vi "TempStringFormatter.vi"(11 "Parsed List":string[](array[string])) -> (3 "string to write":string)   [LabVIEW 2012]
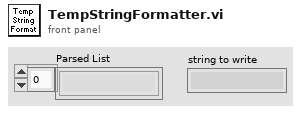
[diagram p1: front panel]
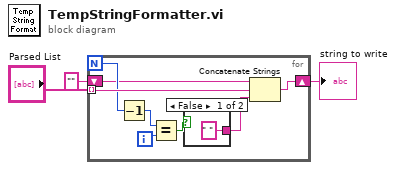
[diagram p0: block diagram]
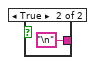
[diagram p2: hidden frame]
diagram:
  n1 = for {
    N -> [w7]
    tunnel: "Parsed List" -> [w10] mode=indexing
    shift-right: [w5] -> w1
    shift-left: "" -> [w4]
    i -> [w9]
    n2 = Decrement(x=w7) -> (x-1=w6:i32)
    n3 = Equal?(x=w6, y=w9) -> (x = y?=w8:bool)
    n4 = case shown="False" w8 {
      tunnel: [" " "\n"] -> w11
      frame False {
      }
      frame True {
      }
    }
    n5 = Concatenate Strings(w4, w10, w11) -> (w5:string)
  }
  "string to write" <- w1
